vi "Git-Get Repo Info by Key.vi"(10 "Repo Info":string[][](array[string]), 11 "Key":string) -> (3 "<JSON>":string)   [LabVIEW 2020]
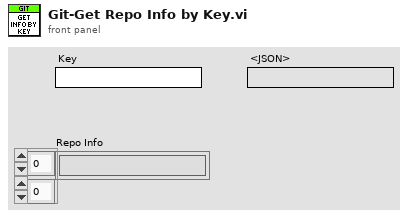
[diagram p1: front panel]
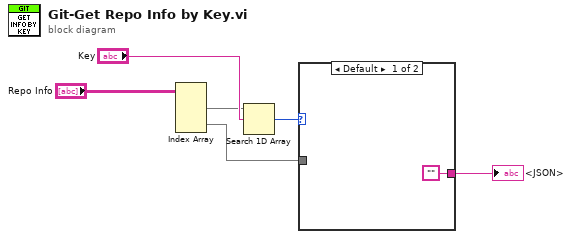
[diagram p0: block diagram]
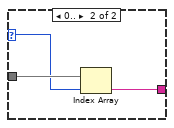
[diagram p2: hidden frame]
diagram:
  n1 = Index Array(array="Repo Info") -> (element #1=w1:string[], element #2=w5:string[])  [unwired: 4 in]
  n2 = Search 1D Array(1D array=w1, element="Key") -> (index of element=w4:i32)  [unwired: 1 in]
  n3 = case shown="Default" w4 {
    selector: w4 -> [_ w9]
    tunnel: w5 -> [_ w10]
    tunnel: ["" ("<JSON>") w8] -> w6
    frame Default {
    }
    frame 0.. {
      n4 = Index Array(array=w10, index=w9) -> (element=w8:string)
    }
  }
  "<JSON>" <- w6
